vi "Complex SVD Decomposition.vi"(9 "SVD option":T2 items=["Thin", "Full"], 10 "singular values only?":bool, 11 "A":T1) -> (0 "error":i32, 1 "Matrix V":T1, 2 "Matrix S":T1, 3 "Matrix U":T1, 5 "Vector S":dbl[](array[numeric]))   [LabVIEW 2017, in "NI_AALPro.lvlib"]
doc: "Computes the singular value decomposition (SVD) of the m x n matrix <B>A</B>. Wire data to the <B>A</B> input to determine the polymorphic instance to use or manually select the instance."
uses:
  NI_AALPro.lvlib
  ComplexMatrix.ctl
  SVD Option.ctl
  <resource>/lvanlys.dll
  NI_Matrix.lvlib
panel:
  # "Complex SVD Decomposition"
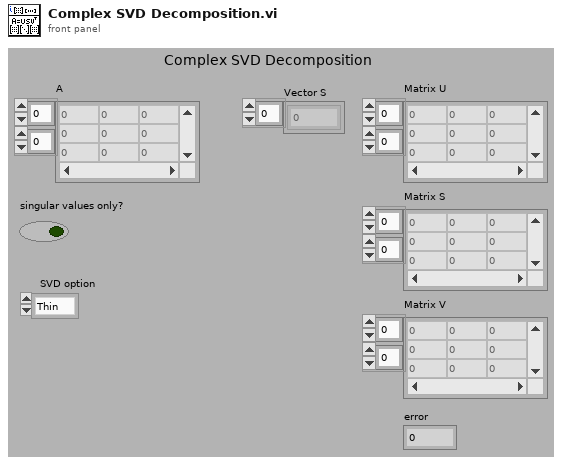
[diagram p1: front panel]
types:
  T1 = typedef "NI_Matrix.lvlib/ComplexMatrix.ctl" = cdb[][]
  T2 = typedef "NI_AALPro.lvlib/SVD Option.ctl" = u16
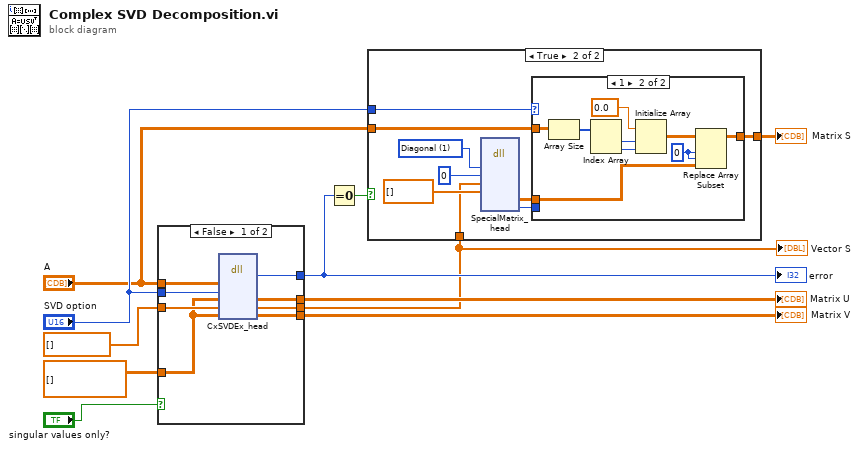
[diagram p0: block diagram]
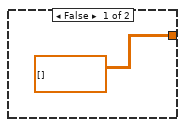
[diagram p2: hidden frame]
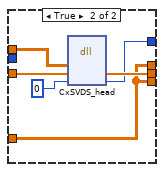
[diagram p4: hidden frame]
diagram:
  n1 = case shown="False" "singular values only?" {
    tunnel: [w19 w21] -> w11
    tunnel: [w18 w21] -> w10
    tunnel: [w17 w20] -> w2
    tunnel: dbl[] [] ("S") -> [w16 w24]
    tunnel: "SVD option" -> [w15 _]
    tunnel: [w14 w22] -> w1
    tunnel: "A" -> [w13 w25]
    tunnel: cdb[][] [] ("S") -> [w12 w21]
    frame False {
      n2 = dll-call lib="C:/Program Files (x86)/National Instruments/LabVIEW 2017/resource/lvanlys.*" fn="CxSVDEx_head"("aH"=w13, "flag"=w15, "uH"=w12, "sH"=w16, "vH"=w12) -> ("return type"=w17:i32, "uH"=w19:cdb[][], "sH"=w14:dbl[], "vH"=w18:cdb[][])  [unwired: 5 in, 2 out]
    }
    frame True {
      n3 = dll-call lib="C:/Program Files (x86)/National Instruments/LabVIEW 2017/resource/lvanlys.*" fn="CxSVDS_head"("A"=w25, "S"=w24, "input param"=0) -> ("S"=w22:dbl[], "input param"=w20:i32)  [unwired: 5 in, 2 out]
    }
  }
  "Matrix U" <- w11
  "Matrix V" <- w10
  "error" <- w2
  "Vector S" <- w1
  n4 = Equal To 0?(x=w2) -> (x = 0?=w3:bool)
  n5 = case shown="True" w3 {
    tunnel: "SVD option" -> [_ w35]
    tunnel: w1 -> [_ w28]
    tunnel: [T1 [] ("Matrix S") w34] -> w7
    tunnel: "A" -> [_ w33]
    frame False {
    }
    frame True {
      w30 = 1 items=["Identity", "Diagonal", "Toepliz", "Vandermonde", "Companion", "Hankel", "Hadamard", "Wilkinson", "Hilbert", "Inverse Hilbert", "Rosser", "Pascal"] ("matrix type")
      n6 = dll-call lib="C:/Program Files (x86)/National Instruments/LabVIEW 2017/resource/lvanlys.*" fn="SpecialMatrix_head"("mtype"=w30, "msize"=0 ("matrix size"), "v1H"=w28, "v2H"=dbl[] [] ("S")) -> ("aH"=w29:dbl[][], "dsperr"=w27:i32)  [unwired: 10 in, 2 out]
      n7 = case shown="1" w35 {
        tunnel: [w36 w38] -> w34
        tunnel: w33 -> [_ w42]
        tunnel: w29 -> [w36 w37]
        tunnel: w27 -> [_ _]
        frame 0, Default {
        }
        frame 1 {
          w39 = 0 ("index (row)")
          n8 = Array Size(array=w42) -> (size(s)=w41:i32[])
          n9 = Index Array(array=w41) -> (element #1=w44:i32, element #2=w43:i32)  [unwired: 2 in]
          n10 = Initialize Array(0.0 ("element"), w44, w43) -> (w40:dbl[][])
          n11 = Replace Array Subset(array=w40, new element=w37, index (row)=w39, index (col)=w39) -> (w38:dbl[][])
        }
      }
    }
  }
  "Matrix S" <- w7
